vi "white line 3.vi"   [LabVIEW 2010, in "Line Follower.lvrbt"]
uses:
  Line Follower.lvrbt
  <vilib>/NXT/Block Support/NXT_InputPort.ctl
  <vilib>/NXT/Subs/MotorOutput.ctl
  <vilib>/NXT/Dual Mode Library/Sensors/Light_On.vi
  <vilib>/NXT/Dual Mode Library/Display/drawNumber.vi
  <vilib>/NXT/Dual Mode Library/Waits/Wait_Num(msec).vi
  <vilib>/NXT/Dual Mode Library/Motors/MotorOn.vi
  <vilib>/NXT/Dual Mode Library/Motors/MotorBrake.vi
  <vilib>/NXT/Dual Mode Library/Sound/Tone.vi
  <vilib>/NXT/Dual Mode Library/Sensors/Sonar_cm.vi
types:
  T1 = typedef "NXT_InputPort.ctl" = u8
  T2 = typedef "LVHSConnector.ctl" = cluster{"Hardware":string, "Flattened String":string}
  T3 = typedef "MotorOutput.ctl" = u8
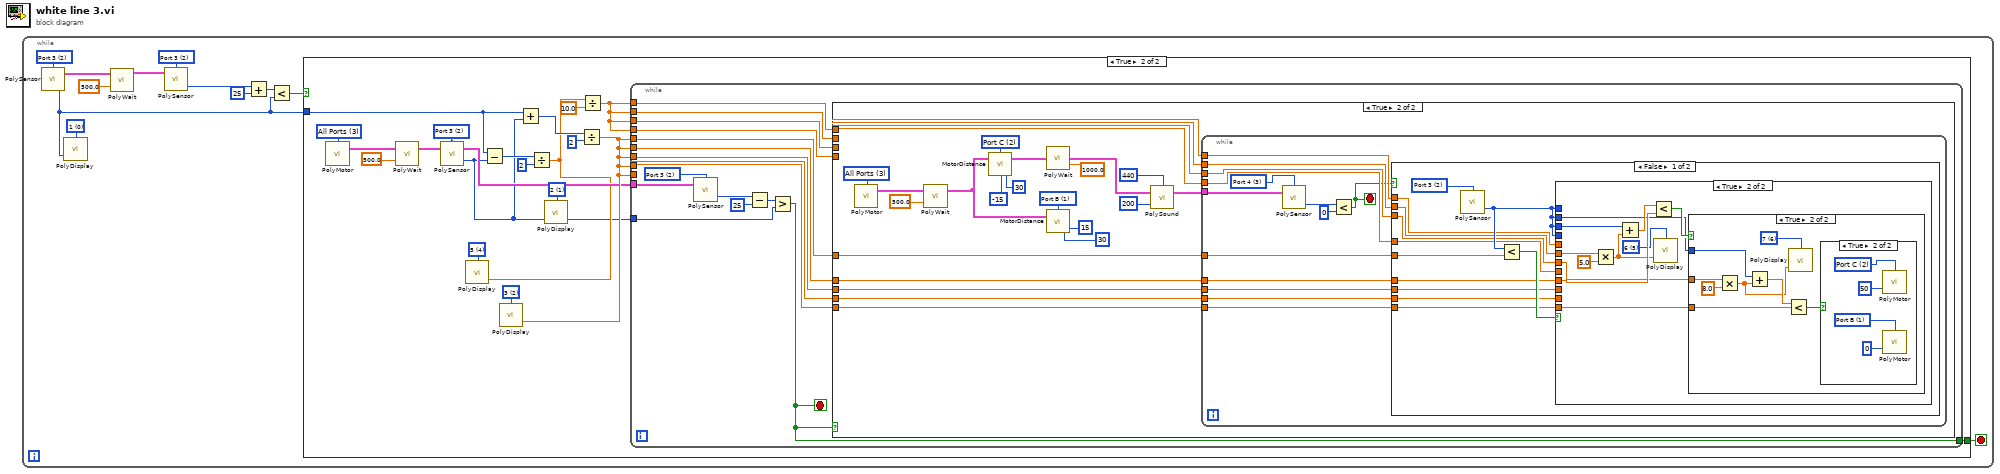
[diagram p0: block diagram]
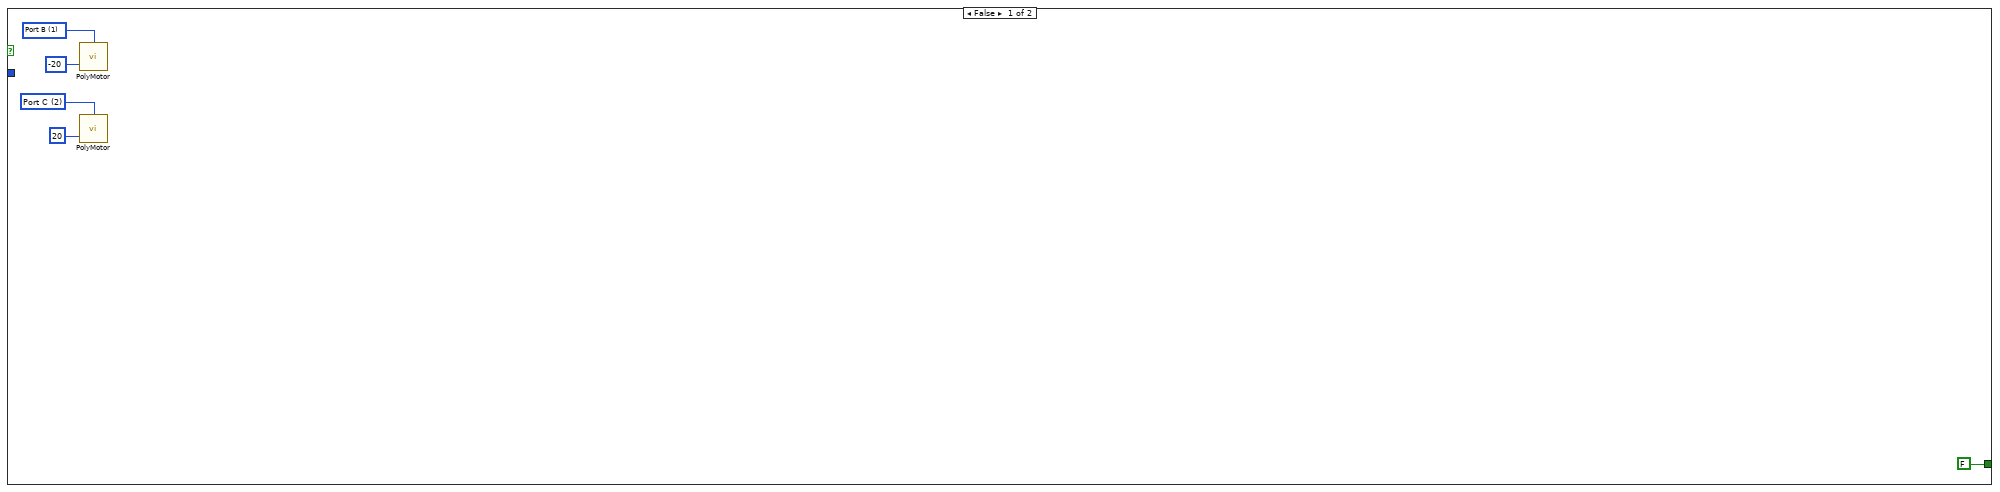
[diagram p2: hidden frame]
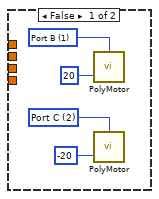
[diagram p3: hidden frame]
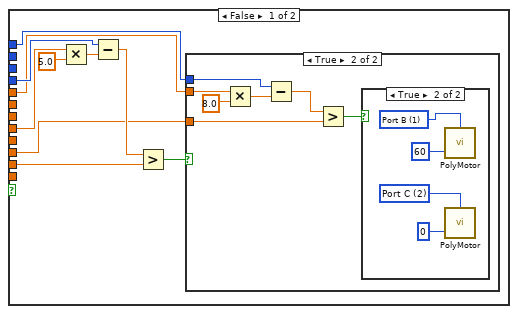
[diagram p4: hidden frame]
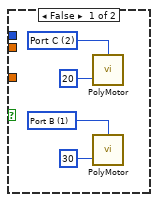
[diagram p5: hidden frame]
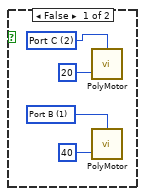
[diagram p6: hidden frame]
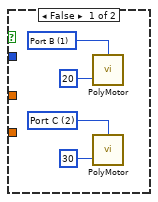
[diagram p7: hidden frame]
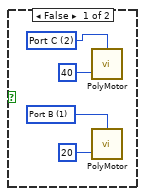
[diagram p8: hidden frame]
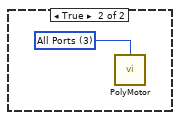
[diagram p9: hidden frame]
diagram:
  n1 = while {
    stop <- w5 stop-if-true
    w3 = T1 2 items=["Port 1", "Port 2", "Port 3", "Port 4"] ("Port (Port 3)")
    w4 = T1 2 items=["Port 1", "Port 2", "Port 3", "Port 4"] ("Port (Port 3)")
    w7 = i16 0 items=["1", "2", "3", "4", "5", "6", "7", "8"] ("Line")
    n2 = call-poly <vilib>:"PolySensor.vi"("Port (Port 3)"=w3) -> ("Scaled Value"=w1:i16, "NXT"=w9:T2)  [unwired: 2 in]
    n3 = call-poly <vilib>:"PolyDisplay.vi"("number"=w1, "Line"=w7) -> ()  [unwired: 2 in, 1 out]
    n4 = call-poly <vilib>:"PolyWait.vi"("Time (100 msec)"=sgl 500.0 ("Time (1 sec)"), "NXT"=w9) -> ("NXT"=w2:T2)  [unwired: 2 in]
    n5 = call-poly <vilib>:"PolySensor.vi"("NXT"=w2, "Port (Port 3)"=w4) -> ("Scaled Value"=w11:i16)  [unwired: 1 in, 1 out]
    n6 = Add(x=w11, y=i16 25) -> (x+y=w6:i16)
    n7 = Less?(x=w6, y=w1) -> (x < y?=w10:bool)
    n8 = case shown="True" w10 {
      tunnel: w1 -> [_ w18]
      tunnel: [FALSE w31] -> w5
      frame False {
        w15 = T3 1 items=["Port A"=0, "Port B"=1, "Port C"=2, "Ports A & B"=4, "Ports A & C"=5, "Ports B & C"=6, "All Ports"=3] ("Port (All Ports)")
        w17 = T3 2 items=["Port A"=0, "Port B"=1, "Port C"=2, "Ports A & B"=4, "Ports A & C"=5, "Ports B & C"=6, "All Ports"=3] ("Output Port (All Ports)")
        n9 = call-poly <vilib>:"PolyMotor.vi"("Power (75)"=-20, "Output Port (All Ports)"=w15) -> ()  [unwired: 2 in, 1 out]
        n10 = call-poly <vilib>:"PolyMotor.vi"("Power (75)"=20, "Output Port (All Ports)"=w17) -> ()  [unwired: 2 in, 1 out]
      }
      frame True {
        w19 = T1 2 items=["Port 1", "Port 2", "Port 3", "Port 4"] ("Port (Port 3)")
        w21 = i16 4 items=["1", "2", "3", "4", "5", "6", "7", "8"] ("Line")
        w33 = i16 1 items=["1", "2", "3", "4", "5", "6", "7", "8"] ("Line")
        w34 = i16 2 items=["1", "2", "3", "4", "5", "6", "7", "8"] ("Line")
        w37 = T3 3 items=["Port A"=0, "Port B"=1, "Port C"=2, "Ports A & B"=4, "Ports A & C"=5, "Ports B & C"=6, "All Ports"=3] ("Port (All Ports)")
        n11 = call-poly <vilib>:"PolyMotor.vi"("Port (All Ports)"=w37) -> ("NXT"=w29:T2)  [unwired: 3 in]
        n12 = call-poly <vilib>:"PolyWait.vi"("Time (100 msec)"=sgl 500.0 ("Time (1 sec)"), "NXT"=w29) -> ("NXT"=w28:T2)  [unwired: 2 in]
        n13 = call-poly <vilib>:"PolySensor.vi"("NXT"=w28, "Port (Port 3)"=w19) -> ("Scaled Value"=w20:i16, "NXT"=w27:T2)  [unwired: 1 in]
        n14 = Subtract(x=w18, y=w20) -> (x-y=w26:i16)
        n15 = Add(x=w18, y=w20) -> (x+y=w35:i16)
        n16 = Divide(x=w26, y=i16 2) -> (x/y=w22:dbl)
        n17 = call-poly <vilib>:"PolyDisplay.vi"("number"=w22, "Line"=w21) -> ()  [unwired: 2 in, 1 out]
        n18 = call-poly <vilib>:"PolyDisplay.vi"("number"=w20, "Line"=w33) -> ()  [unwired: 2 in, 1 out]
        n19 = Divide(x=w35, y=i16 2) -> (x/y=w30:dbl)
        n20 = call-poly <vilib>:"PolyDisplay.vi"("number"=w30, "Line"=w34) -> ()  [unwired: 2 in, 1 out]
        n21 = Divide(x=w22, y=10.0) -> (x/y=w23:dbl)
        n22 = while {
          tunnel: w20 -> [w51]
          tunnel: w30 -> [w49]
          tunnel: w30 -> [w48]
          tunnel: w30 -> [w45]
          tunnel: w27 -> [w47]
          tunnel: [w46] -> w31
          tunnel: w30 -> [w44]
          tunnel: w30 -> [w43]
          tunnel: w23 -> [w42]
          tunnel: w23 -> [w41]
          tunnel: w23 -> [w40]
          tunnel: w23 -> [w39]
          stop <- w46 stop-if-true
          w38 = T1 2 items=["Port 1", "Port 2", "Port 3", "Port 4"] ("Port (Port 3)")
          n23 = call-poly <vilib>:"PolySensor.vi"("NXT"=w47, "Port (Port 3)"=w38) -> ("Scaled Value"=w52:i16)  [unwired: 1 in, 1 out]
          n24 = Subtract(x=w52, y=i16 25) -> (x-y=w50:i16)
          n25 = Greater?(x=w50, y=w51) -> (0:w46:bool)
          n26 = case shown="True" w46 {
            tunnel: w49 -> [_ w71]
            tunnel: w48 -> [_ w70]
            tunnel: w45 -> [_ w69]
            tunnel: w44 -> [_ w66]
            tunnel: w43 -> [_ w65]
            tunnel: w42 -> [_ w61]
            tunnel: w41 -> [_ w60]
            tunnel: w40 -> [_ w59]
            tunnel: w39 -> [_ w58]
            frame False {
              w55 = T3 2 items=["Port A"=0, "Port B"=1, "Port C"=2, "Ports A & B"=4, "Ports A & C"=5, "Ports B & C"=6, "All Ports"=3] ("Port (All Ports)")
              w57 = T3 1 items=["Port A"=0, "Port B"=1, "Port C"=2, "Ports A & B"=4, "Ports A & C"=5, "Ports B & C"=6, "All Ports"=3] ("Output Port (All Ports)")
              n27 = call-poly <vilib>:"PolyMotor.vi"("Power (75)"=20, "Output Port (All Ports)"=w57) -> ()  [unwired: 2 in, 1 out]
              n28 = call-poly <vilib>:"PolyMotor.vi"("Power (75)"=-20, "Output Port (All Ports)"=w55) -> ()  [unwired: 2 in, 1 out]
            }
            frame True {
              w79 = T3 2 items=["Port A"=0, "Port B"=1, "Port C"=2, "Ports A & B"=4, "Ports A & C"=5, "Ports B & C"=6, "All Ports"=3] ("Port (All Ports)")
              w77 = T3 1 items=["Port A"=0, "Port B"=1, "Port C"=2, "Ports A & B"=4, "Ports A & C"=5, "Ports B & C"=6, "All Ports"=3] ("Output Port (All Ports)")
              w82 = T3 3 items=["Port A"=0, "Port B"=1, "Port C"=2, "Ports A & B"=4, "Ports A & C"=5, "Ports B & C"=6, "All Ports"=3] ("Port (All Ports)")
              n29 = call-poly <vilib>:"PolyMotor.vi"("Port (All Ports)"=w82) -> ("NXT"=w72:T2)  [unwired: 3 in]
              n30 = call-poly <vilib>:"PolyWait.vi"("Time (100 msec)"=sgl 500.0 ("Time (1 sec)"), "NXT"=w72) -> ("NXT"=w74:T2)  [unwired: 2 in]
              n31 = call <vilib>:"MotorDistance.vi"("Power (75)"=-15, "Angle of Rotation (360)"=30, "NXT"=w74, "Output Port (All Ports)"=w79) -> ("NXT"=w64:T2)
              n32 = call-poly <vilib>:"PolyWait.vi"("Time (100 msec)"=sgl 1000.0 ("Time (1 sec)"), "NXT"=w64) -> ("NXT"=w63:T2)  [unwired: 2 in]
              n33 = call <vilib>:"MotorDistance.vi"("Power (75)"=15, "Angle of Rotation (360)"=30, "NXT"=w74, "Output Port (All Ports)"=w77) -> ()  [unwired: 1 out]
              n34 = call-poly <vilib>:"PolySound.vi"("Duration (500 ms)"=u16 200, "NXT"=w63, "Tone (440 Hz)"=u16 440) -> ("NXT"=w62:T2)  [unwired: 1 in]
              n35 = while {
                tunnel: w62 -> [w94]
                tunnel: w71 -> [w93]
                tunnel: w70 -> [w92]
                tunnel: w69 -> [w91]
                tunnel: w66 -> [w90]
                tunnel: w65 -> [w89]
                tunnel: w61 -> [w88]
                tunnel: w60 -> [w87]
                tunnel: w59 -> [w86]
                tunnel: w58 -> [w85]
                stop <- w83 stop-if-true
                w96 = T1 3 items=["Port 1", "Port 2", "Port 3", "Port 4"] ("Port (Port 4)")
                n36 = call-poly <vilib>:"PolySensor.vi"("NXT"=w94, "Port (Port 4)"=w96) -> ("Distance (cm)"=w84:i16)  [unwired: 1 in, 1 out]
                n37 = Less?(x=w84, y=i16 0) -> (x < y?=w83:bool)
                n38 = case shown="False" w83 {
                  tunnel: w93 -> [w107 _]
                  tunnel: w92 -> [w106 _]
                  tunnel: w91 -> [w105 _]
                  tunnel: w90 -> [w104 _]
                  tunnel: w89 -> [w102 _]
                  tunnel: w88 -> [w101 _]
                  tunnel: w87 -> [w100 _]
                  tunnel: w86 -> [w99 _]
                  tunnel: w85 -> [w98 _]
                  frame False {
                    w97 = T1 2 items=["Port 1", "Port 2", "Port 3", "Port 4"] ("Port (Port 3)")
                    n39 = call-poly <vilib>:"PolySensor.vi"("Port (Port 3)"=w97) -> ("Scaled Value"=w103:i16)  [unwired: 2 in, 1 out]
                    n40 = Less?(x=w103, y=w107) -> (x < y?=w108:bool)
                    n41 = case shown="True" w108 {
                      tunnel: w103 -> [w116 _]
                      tunnel: w103 -> [_ w146]
                      tunnel: w106 -> [w115 _]
                      tunnel: w105 -> [_ w145]
                      tunnel: w103 -> [w114 _]
                      tunnel: w104 -> [w113 _]
                      tunnel: w103 -> [_ w144]
                      tunnel: w102 -> [_ w143]
                      tunnel: w101 -> [_ w141]
                      tunnel: w100 -> [_ w140]
                      tunnel: w99 -> [w111 _]
                      tunnel: w98 -> [w110 _]
                      frame False {
                        n42 = Multiply(x=w111, y=5.0) -> (x*y=w109:dbl)
                        n43 = Subtract(x=w116, y=w109) -> (x-y=w117:dbl)
                        n44 = Greater?(x=w117, y=w115) -> (0:w118:bool)
                        n45 = case shown="True" w118 {
                          tunnel: w114 -> [_ w129]
                          tunnel: w113 -> [_ w127]
                          tunnel: w110 -> [_ w124]
                          frame False {
                            w121 = T3 2 items=["Port A"=0, "Port B"=1, "Port C"=2, "Ports A & B"=4, "Ports A & C"=5, "Ports B & C"=6, "All Ports"=3] ("Port (All Ports)")
                            w119 = T3 1 items=["Port A"=0, "Port B"=1, "Port C"=2, "Ports A & B"=4, "Ports A & C"=5, "Ports B & C"=6, "All Ports"=3] ("Output Port (All Ports)")
                            n46 = call-poly <vilib>:"PolyMotor.vi"("Power (75)"=20, "Output Port (All Ports)"=w121) -> ()  [unwired: 2 in, 1 out]
                            n47 = call-poly <vilib>:"PolyMotor.vi"("Power (75)"=30, "Output Port (All Ports)"=w119) -> ()  [unwired: 2 in, 1 out]
                          }
                          frame True {
                            n48 = Multiply(x=w124, y=8.0) -> (x*y=w123:dbl)
                            n49 = Subtract(x=w129, y=w123) -> (x-y=w128:dbl)
                            n50 = Greater?(x=w128, y=w127) -> (0:w126:bool)
                            n51 = case shown="True" w126 {
                              frame False {
                                w132 = T3 2 items=["Port A"=0, "Port B"=1, "Port C"=2, "Ports A & B"=4, "Ports A & C"=5, "Ports B & C"=6, "All Ports"=3] ("Port (All Ports)")
                                w130 = T3 1 items=["Port A"=0, "Port B"=1, "Port C"=2, "Ports A & B"=4, "Ports A & C"=5, "Ports B & C"=6, "All Ports"=3] ("Output Port (All Ports)")
                                n52 = call-poly <vilib>:"PolyMotor.vi"("Power (75)"=20, "Output Port (All Ports)"=w132) -> ()  [unwired: 2 in, 1 out]
                                n53 = call-poly <vilib>:"PolyMotor.vi"("Power (75)"=40, "Output Port (All Ports)"=w130) -> ()  [unwired: 2 in, 1 out]
                              }
                              frame True {
                                w136 = T3 2 items=["Port A"=0, "Port B"=1, "Port C"=2, "Ports A & B"=4, "Ports A & C"=5, "Ports B & C"=6, "All Ports"=3] ("Port (All Ports)")
                                w134 = T3 1 items=["Port A"=0, "Port B"=1, "Port C"=2, "Ports A & B"=4, "Ports A & C"=5, "Ports B & C"=6, "All Ports"=3] ("Output Port (All Ports)")
                                n54 = call-poly <vilib>:"PolyMotor.vi"("Power (75)"=60, "Output Port (All Ports)"=w134) -> ()  [unwired: 2 in, 1 out]
                                n55 = call-poly <vilib>:"PolyMotor.vi"("Power (75)"=0, "Output Port (All Ports)"=w136) -> ()  [unwired: 2 in, 1 out]
                              }
                            }
                          }
                        }
                      }
                      frame True {
                        w138 = i16 5 items=["1", "2", "3", "4", "5", "6", "7", "8"] ("Line")
                        n56 = Multiply(x=w141, y=5.0) -> (x*y=w139:dbl)
                        n57 = Add(x=w146, y=w139) -> (x+y=w148:dbl)
                        n58 = Less?(x=w148, y=w145) -> (x < y?=w147:bool)
                        n59 = call-poly <vilib>:"PolyDisplay.vi"("number"=w139, "Line"=w138) -> ()  [unwired: 2 in, 1 out]
                        n60 = case shown="True" w147 {
                          tunnel: w144 -> [_ w160]
                          tunnel: w143 -> [_ w159]
                          tunnel: w140 -> [_ w155]
                          frame False {
                            w152 = T3 1 items=["Port A"=0, "Port B"=1, "Port C"=2, "Ports A & B"=4, "Ports A & C"=5, "Ports B & C"=6, "All Ports"=3] ("Port (All Ports)")
                            w150 = T3 2 items=["Port A"=0, "Port B"=1, "Port C"=2, "Ports A & B"=4, "Ports A & C"=5, "Ports B & C"=6, "All Ports"=3] ("Output Port (All Ports)")
                            n61 = call-poly <vilib>:"PolyMotor.vi"("Power (75)"=20, "Output Port (All Ports)"=w152) -> ()  [unwired: 2 in, 1 out]
                            n62 = call-poly <vilib>:"PolyMotor.vi"("Power (75)"=30, "Output Port (All Ports)"=w150) -> ()  [unwired: 2 in, 1 out]
                          }
                          frame True {
                            w153 = i16 6 items=["1", "2", "3", "4", "5", "6", "7", "8"] ("Line")
                            n63 = Multiply(x=w155, y=8.0) -> (x*y=w154:dbl)
                            n64 = Add(x=w160, y=w154) -> (x+y=w158:dbl)
                            n65 = Less?(x=w158, y=w159) -> (x < y?=w157:bool)
                            n66 = call-poly <vilib>:"PolyDisplay.vi"("number"=w154, "Line"=w153) -> ()  [unwired: 2 in, 1 out]
                            n67 = case shown="True" w157 {
                              frame False {
                                w163 = T3 1 items=["Port A"=0, "Port B"=1, "Port C"=2, "Ports A & B"=4, "Ports A & C"=5, "Ports B & C"=6, "All Ports"=3] ("Port (All Ports)")
                                w161 = T3 2 items=["Port A"=0, "Port B"=1, "Port C"=2, "Ports A & B"=4, "Ports A & C"=5, "Ports B & C"=6, "All Ports"=3] ("Output Port (All Ports)")
                                n68 = call-poly <vilib>:"PolyMotor.vi"("Power (75)"=40, "Output Port (All Ports)"=w161) -> ()  [unwired: 2 in, 1 out]
                                n69 = call-poly <vilib>:"PolyMotor.vi"("Power (75)"=20, "Output Port (All Ports)"=w163) -> ()  [unwired: 2 in, 1 out]
                              }
                              frame True {
                                w166 = T3 1 items=["Port A"=0, "Port B"=1, "Port C"=2, "Ports A & B"=4, "Ports A & C"=5, "Ports B & C"=6, "All Ports"=3] ("Port (All Ports)")
                                w165 = T3 2 items=["Port A"=0, "Port B"=1, "Port C"=2, "Ports A & B"=4, "Ports A & C"=5, "Ports B & C"=6, "All Ports"=3] ("Output Port (All Ports)")
                                n70 = call-poly <vilib>:"PolyMotor.vi"("Power (75)"=50, "Output Port (All Ports)"=w165) -> ()  [unwired: 2 in, 1 out]
                                n71 = call-poly <vilib>:"PolyMotor.vi"("Power (75)"=0, "Output Port (All Ports)"=w166) -> ()  [unwired: 2 in, 1 out]
                              }
                            }
                          }
                        }
                      }
                    }
                  }
                  frame True {
                    w169 = T3 3 items=["Port A"=0, "Port B"=1, "Port C"=2, "Ports A & B"=4, "Ports A & C"=5, "Ports B & C"=6, "All Ports"=3] ("Port (All Ports)")
                    n72 = call-poly <vilib>:"PolyMotor.vi"("Port (All Ports)"=w169) -> ()  [unwired: 3 in, 1 out]
                  }
                }
              }
            }
          }
        }
      }
    }
  }
